vi "createForceAndStatusFrame.vi"(8 "error in (no error)":errorcluster, 9 "TriggerIRQ":bool, 10 "WaitForTrigger":bool, 11 "HardPointActuator in":refnum<class "HPILC.lvclass">) -> (0 "error out":errorcluster, 2 "Frame":T1 {"Data" format="%02x"}, 3 "HardPointActuator out":refnum<class "HPILC.lvclass">)   [LabVIEW 2015, in "RTHPILC.lvlib" / "HPILC.lvclass"]
uses:
  HPILC.lvclass
  Common_RT_Modbus/DataTypes/Frame.ctl
  Common_RT_Modbus/DynamicFrameBuilder/DynamicFrameBuilder.lvclass
  Common_RT_ILC/ILC/ILC.lvclass/ILC.ctl
  Common_RT_ILC/ILC/ILC.lvclass
  Common_RT_Modbus/RTModbus.lvlib
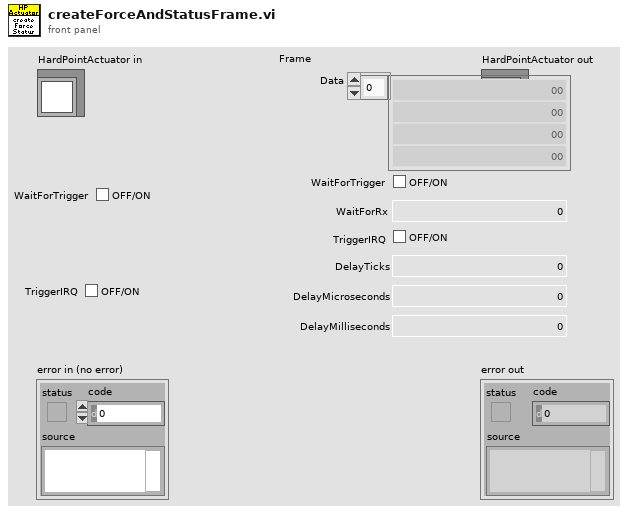
[diagram p1: front panel]
types:
  T1 = typedef "RTModbus.lvlib/Frame.ctl" = cluster{"Data":u8[], "WaitForTrigger":bool, "WaitForRx":u16, "TriggerIRQ":bool, "DelayTicks":u16, "DelayMicroseconds":u16, "DelayMilliseconds":u16}
  T2 = typedef "RTILC.lvlib/ILCData.ctl" = cluster{"Constants":T3, "Command":T4, "Telemetry":T5, "Responses":T6}
  T3 = typedef "RTILC.lvlib/ILCConstants.ctl" = cluster{"Subnet":u8, "Address":u8}
  T4 = typedef "RTILC.lvlib/ILCCommand.ctl" = cluster{"ILCMode":u16, "TemporaryAddress":u8}
  T5 = typedef "RTILC.lvlib/ILCTelemetry.ctl" = cluster{"UniqueID":u64, "FirmwareType":u8, "NetworkNodeType":u8, "ILCOption":u8, "NetworkNodeOption":u8, "MajorRevision":u8, "MinorRevision":u8, "FirmwareName":string, "ILCMode":u16, "MajorFault":bool, "MinorFault":bool, "FaultOverride":bool, "UniqueIDCRCMismatch":bool, "AppTypeNodeTypeMismatch":bool, "AppMissing":bool, "AppCRCMismatch":bool, "TEDSNotFound":bool, "TEDS1Mismatch":bool, "TEDS2Mismatch":bool, "WatchdogResetDetected":bool, "BrownoutDetected":bool, "EventTrapResetDetected":bool, "TemporaryAddress":u8}
  T6 = typedef "RTILC.lvlib/ILCResponses.ctl" = cluster{"ReportServerID":T7, "ReportServerStatus":T7, "ILCMode":T7, "SetTemporaryAddress":T7, "Reset":T7}
  T7 = typedef "RTModbus.lvlib/ExceptionCodes.ctl" = enum16{"None", "IllegalFunction", "IllegalDataAddress", "IllegalDataValue", "SlaveDeviceFailure", "Acknowledge", "SlaveDeviceBusy", "NegativeAcknowledge", "MemoryParityError", "GatewayPathUnavailable", "GatewayTargetDeviceFailedToRespond"}
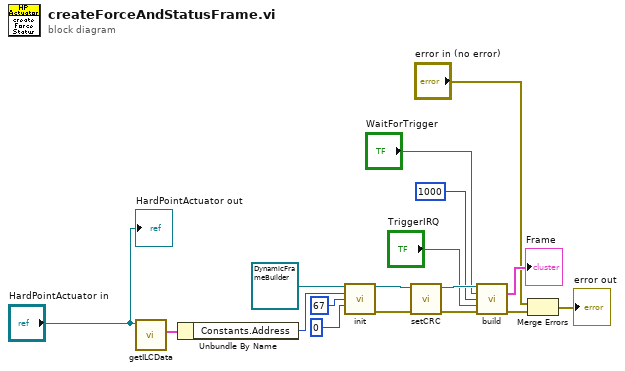
[diagram p0: block diagram]
diagram:
  n1 = call "getILCData.vi"("ILC in"="HardPointActuator in") -> ("ILCData"=w17:T2)  [unwired: 9 in, 1 out]
  n2 = Unbundle By Name(w17) -> ("Constants.Address"=w16:u8)
  n3 = call "init.vi"("DynamicFrameBuilder in"=refnum<class "DynamicFrameBuilder.lvclass"> refnum ("RTModbus.lvlib:DynamicFrameBuilder.lvclass"), "Address"=w16, "Function"=u8 67, "DataSize"=0) -> ("DynamicFrameBuilder out"=w1:refnum<class "DynamicFrameBuilder.lvclass">, "error out"=w2:errorcluster)  [unwired: 10 in]
  n4 = call "setCRC.vi"("error in (no error)"=w2, "DynamicFrameBuilder in"=w1) -> ("error out"=w7:errorcluster, "DynamicFrameBuilder out"=w12:refnum<class "DynamicFrameBuilder.lvclass">)  [unwired: 8 in]
  n5 = call "build.vi"("DynamicFrameBuilder in"=w12, "WaitForTrigger"="WaitForTrigger", "WaitForRxTimeout"=u16 1000, "TriggerIRQ"="TriggerIRQ", "error in (no error)"=w7) -> ("Frame"=→"Frame":T1, "error out"=w10:errorcluster)  [unwired: 8 in, 1 out]
  n6 = Merge Errors("error in (no error)", w10) -> (→"error out":errorcluster)
  "HardPointActuator out" <- "HardPointActuator in"
